vi "PluginsLoaderService_GetAvailablePluginsEvent.vi"(8 "error in (no error)":errorcluster, 11 "PluginsLoaderService in":refnum<class "PluginsLoaderService.lvclass">) -> (0 "error out":errorcluster, 2 "AvailablePluginsEvent":refnum<user-event>, 3 "PluginsLoaderService out":refnum<class "PluginsLoaderService.lvclass">)   [LabVIEW 2014, in "PluginsThread.lvlib" / "PluginsLoaderService.lvclass"]
uses:
  PluginsLoaderService.lvclass
  _Plugins/GCMPlugin/GCMPlugin.lvclass
  PluginsLoaderService.lvclass/PluginsLoaderService.ctl
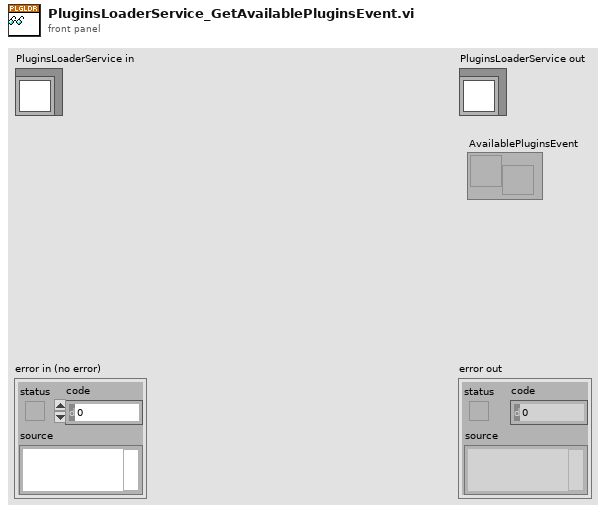
[diagram p1: front panel]
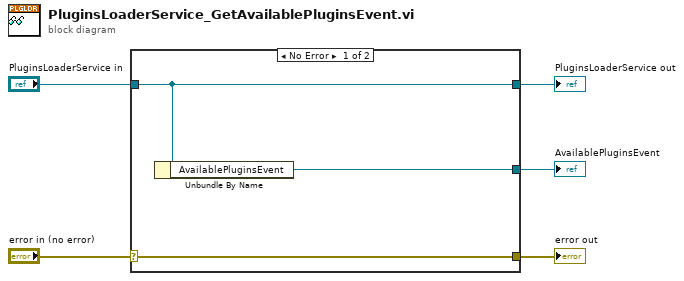
[diagram p0: block diagram]
diagram:
  n1 = case shown="No Error" "error in (no error)" {
    selector: "error in (no error)" -> [w8 w9]
    tunnel: [w8 w9] -> w4
    tunnel: [w7 w10] -> w2
    tunnel: "PluginsLoaderService in" -> [w7 w10]
    tunnel: [w6 _] -> w1
    frame No Error {
      n2 = Unbundle By Name(w7) -> ("AvailablePluginsEvent"=w6:refnum<user-event>)
    }
    frame Error {
    }
  }
  "error out" <- w4
  "PluginsLoaderService out" <- w2
  "AvailablePluginsEvent" <- w1
